vi "Queue COMM Dequeue.vi"(8 "error in (no error)":errorcluster) -> (0 "error out":errorcluster, 3 "element":T1)   [LabVIEW 2026, in "Display.lvlib"]
doc: "For named purposes"
uses:
  Display.lvlib
  Private Control/Queue Element.ctl
  Private Control/Module Action.ctl
  Private Control/Queue FGV Action.ctl
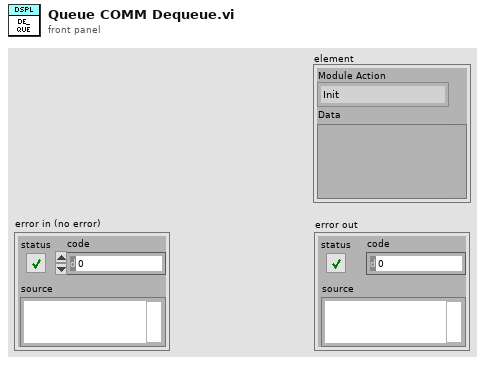
[diagram p1: front panel]
types:
  T1 = typedef "Display.lvlib/Queue Element.ctl" = cluster{"Module Action":T2, "Data":variant}
  T2 = typedef "Display.lvlib/Module Action.ctl" = enum16{"Init", "Error", "Exit"}
  T3 = typedef "Display.lvlib/Queue FGV Action.ctl" = enum16{"Create", "Get", "Release"}
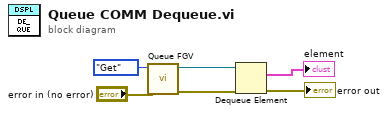
[diagram p0: block diagram]
diagram:
  n1 = call "Queue FGV.vi"("error in (no error)"="error in (no error)", "Queue FGV  Action"=Queue_FGV_Action."Get") -> ("error out"=w4:errorcluster, "queue out"=w3:refnum<queue>)  [unwired: 8 in]
  n2 = Dequeue Element(queue=w3, error in (no error)=w4) -> (element=→"element":T1, error out=→"error out":errorcluster)  [unwired: 1 in, 2 out]
